vi "Initialize UI.vi"(11 "Car Position Simulator in":refnum<class "Car Position Simulator.lvclass">) -> (3 "Car Position Simulator out":refnum<class "Car Position Simulator.lvclass">)   [LabVIEW 2016, in "CLD Exam - Car Wash.lvlib" / "Car Position Simulator.lvclass"]
uses:
  Car Position Simulator.lvclass
  Car Position Simulator.lvclass/Car Position Simulator.ctl
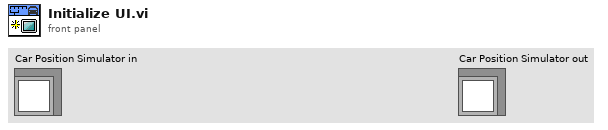
[diagram p1: front panel]
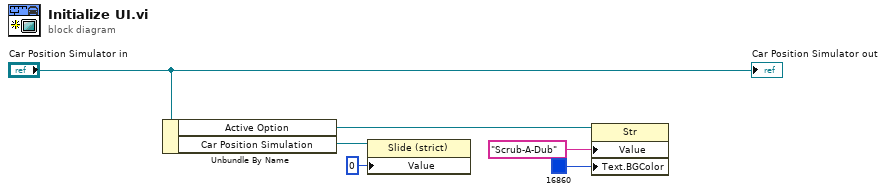
[diagram p0: block diagram]
diagram:
  n1 = Unbundle By Name("Car Position Simulator in") -> ("Active Option"=w3:refnum<vi>, "Car Position Simulation"=w5:refnum<vi>)
  n2 = property class="Slide (strict)"(reference=w5, "Value"=0) -> ()  [unwired: 1 in, 2 out]
  n3 = property class="Str"(reference=w3, "Value"="Scrub-A-Dub", "Text.BGColor"=u32 16860) -> ()  [unwired: 1 in, 2 out]
  "Car Position Simulator out" <- "Car Position Simulator in"
